vi "Perform Action.vi"(8 "error in":errorcluster, 10 "Input":variant, 11 "AI Voltage DAQmx Cont CFG in":refnum<class "AI Voltage DAQmx Cont CFG.lvclass">) -> (0 "error out":errorcluster, 2 "Output":variant, 3 "AI Voltage DAQmx Cont CFG out":refnum<class "AI Voltage DAQmx Cont CFG.lvclass">)   [LabVIEW 2024, in "AI Voltage DAQmx Cont CFG.lvclass"]
uses:
  AI Voltage DAQmx Cont CFG.lvclass
  AI Voltage DAQmx Cont CFG.lvclass/AI Voltage DAQmx Cont CFG.ctl
  DAQmx Base CFG/DAQmx Base CFG.lvclass
  Buffers/BufferLossless/BufferLossless.lvclass
  D:/git/HAL/HAL/Devices/DAQmx/DAQmx Base CFG/DAQmx Base CFG.lvclass
  D:/git/HAL/HAL/Configurations/CFG JSON/CFG JSON.lvclass
  D:/git/HAL/HAL/Configurations/CFG Base/CFG Base.lvclass
  D:/git/HAL/HAL/Devices/DAQmx/AI/AI Voltage DAQmx Cont CFG/AI Voltage DAQmx Cont CFG.lvclass
  <vilib>/DAQmx/read.llb/DAQmx Read (Analog 1D Wfm NChan NSamp).vi
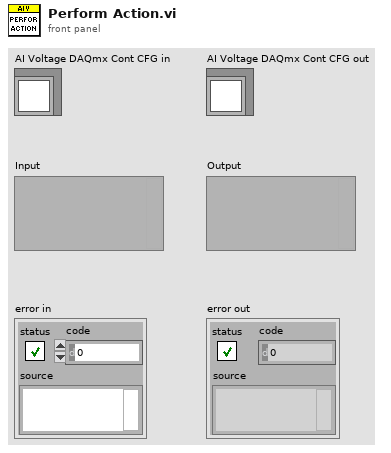
[diagram p1: front panel]
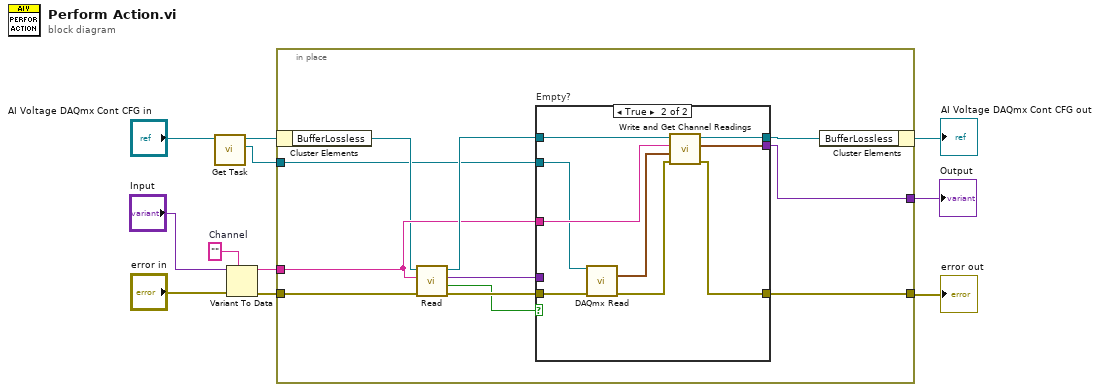
[diagram p0: block diagram]
diagram:
  w11 = ""  # Channel
  n1 = call "Get Task.vi"("DAQmx Base CFG in"="AI Voltage DAQmx Cont CFG in") -> ("Task"=w2:refnum<k21>, "DAQmx Base CFG out"=w3:refnum<class "AI Voltage DAQmx Cont CFG.lvclass">)  [unwired: 9 in]
  n2 = Variant To Data(error in="error in", type=w11, Variant="Input") -> (data=w9:string, error out=w10:errorcluster)
  n3 = in-place {
    in-place-border: w10 -> [w20]
    in-place-border: w9 -> [w19]
    in-place-border: [w18] -> w7
    in-place-border: [w17] -> w5
    in-place-border: w2 -> [w15]
    n4 = in-place-cluster #1(w3) -> ("BufferLossless"=w16:refnum<class "BufferLossless.lvclass">)
    n5 = call "Read.vi"("error in"=w20, "Channel"=w19, "BufferLossless in"=w16) -> ("error out"=w22:errorcluster, "empty?"=w12:bool, "Readings"=w14:variant, "BufferLossless out"=w21:refnum<class "BufferLossless.lvclass">)  [unwired: 5 in]
    n6 = case "Empty?" shown="True" w12 {
      tunnel: [w24 w31] -> w18
      tunnel: w21 -> [w23 w34]
      tunnel: [w25 w28] -> w17
      tunnel: w14 -> [w25 _]
      tunnel: w22 -> [w24 w30]
      tunnel: w19 -> [_ w29]
      tunnel: [w23 w27] -> w13
      tunnel: w15 -> [_ w26]
      frame False {
      }
      frame True {
        n7 = call-poly <vilib>:"DAQmx Read.vi"("task/channels in"=w26, "error in"=w30) -> ("data"=w33:waveform(dbl)[], "error out"=w32:errorcluster)  [unwired: 11 in, 1 out]
        n8 = call "Write and Get Channel Readings.vi"("error in"=w32, "Readings"=w33, "Channel"=w29, "BufferLossless in"=w34) -> ("error out"=w31:errorcluster, "Reading"=w28:waveform(dbl), "BufferLossless out"=w27:refnum<class "BufferLossless.lvclass">)  [unwired: 5 in]
      }
    }
    n9 = in-place-cluster #1("BufferLossless"=w13) -> (→"AI Voltage DAQmx Cont CFG out":refnum<class "AI Voltage DAQmx Cont CFG.lvclass">)
  }
  "error out" <- w7
  "Output" <- w5
